vi "Read Resource.vi"(8 "error in (no error)":errorcluster, 11 "Thermal Camera in":refnum<class "Thermal Camera.lvclass">) -> (0 "error out":errorcluster, 2 "Resource":string, 3 "Thermal Camera out":refnum<class "Thermal Camera.lvclass">)   [LabVIEW 2018, in "Thermal Camera.lvlib" / "Thermal Camera.lvclass"]
uses:
  Thermal Camera.lvclass
  Thermal Camera.lvclass/Thermal Camera.ctl
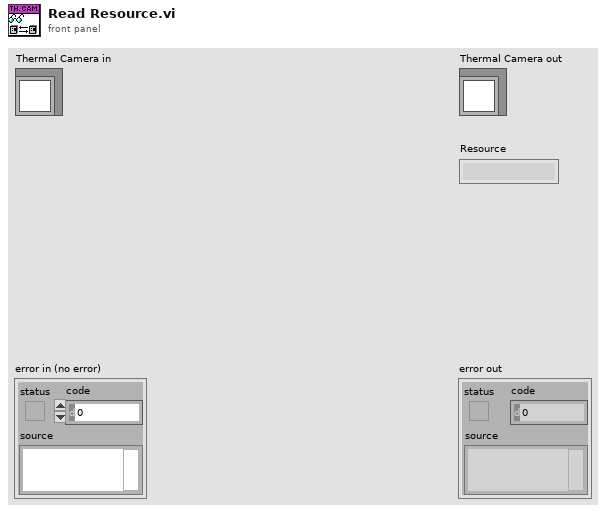
[diagram p1: front panel]
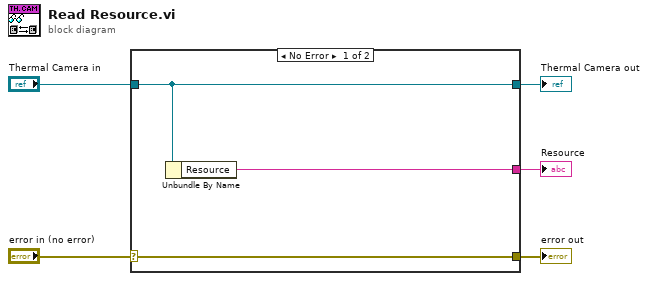
[diagram p0: block diagram]
diagram:
  n1 = case shown="No Error" "error in (no error)" {
    selector: "error in (no error)" -> [w8 w9]
    tunnel: [w8 w9] -> w4
    tunnel: [w7 w10] -> w2
    tunnel: "Thermal Camera in" -> [w7 w10]
    tunnel: [w6 _] -> w1
    frame No Error {
      n2 = Unbundle By Name(w7) -> ("Resource"=w6:string)
    }
    frame Error {
    }
  }
  "error out" <- w4
  "Thermal Camera out" <- w2
  "Resource" <- w1
